vi "Configure Channel.vi"(0 "CS++Scope":refnum<class "CS++Scope.lvclass">, 1 "channel enabled (True)":bool=TRUE, 2 "channel name (\"CHANNEL1\")":string="CHANNEL1", 3 "probe attenuation (1:1.0)":dbl=1.0 format="%.3f", 4 "vertical offset (0.0 V)":dbl[unit] format="%.3f", 5 "error in (no error)":errorcluster, 6 "vertical coupling (DC)":i32(ring)=1 items=["AC", "DC", "GND"], 8 "vertical range (10.0 V)":dbl[unit]=10.0 format="%.3f") -> (14 "CS++Scope out":refnum<class "CS++Scope.lvclass">, 19 "error out":errorcluster)   [LabVIEW 2015, in "CS++Scope.lvlib" / "CS++Scope.lvclass"]
doc: "This VI configures the most commonly configured properties of the oscilloscope channel sub-system. These properties are the range, offset, coupling, probe attenuation, and whether the channel is enabled."
uses:
  CS++Scope.lvclass
  CSPP_Core/Classes/CS++ProcessVariables/ProcessVariable/PV.lvclass
  PV-Enum-n.ctl
  CSPP_Core/Classes/CS++ProcessVariables/ProcessVariable/PV.lvclass/PV.ctl
  CS++Scope.lvclass/CS++Scope.ctl
  CSPP_Core/Classes/CS++ProcessVariables/ProcessVariable/Write Data.vi
  CSPP_Core/Classes/CS++ProcessVariables/ProcessVariable/Write Timestamp.vi
  CSPP_Core/Classes/CS++ProcessVariables/ProcessVariable/Write Quality.vi
  CSPP_Core/Classes/CS++ProcessVariables/ProcessVariable/Write status.vi
  CSPP_Core/Classes/CS++ProcessVariables/PVConnection/PVConnection.lvclass
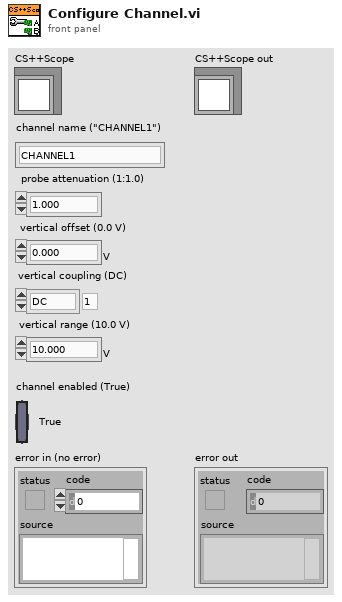
[diagram p1: front panel]
types:
  T1 = typedef "CS++Scope.lvlib/CS++Scope.lvclass/PV-Enum-n.ctl" = enum16{"InputImpedance", "MaxInputFrequency", "VerticalRange", "ProbeAttenuation", "VerticalOffset", "VerticalCoupling", "ChannelEnabled"}
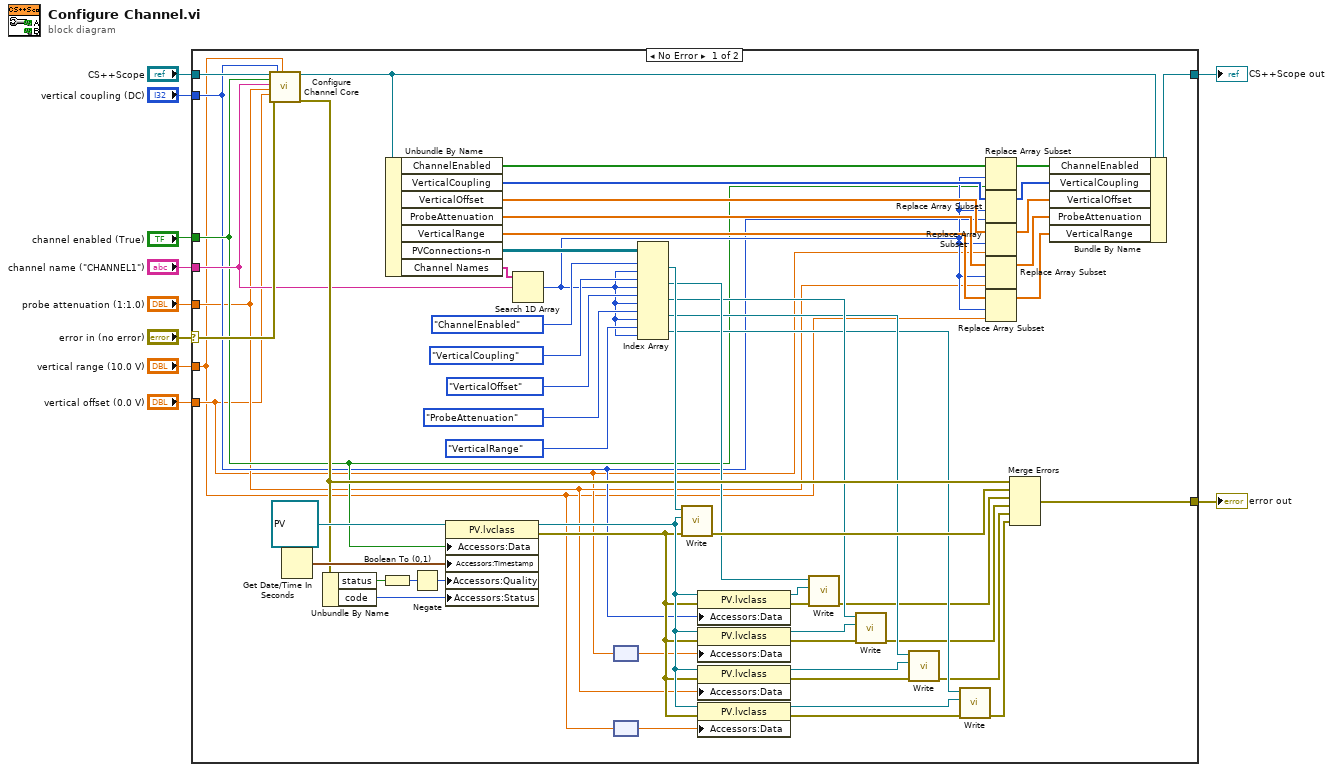
[diagram p0: block diagram]
diagram:
  n1 = case shown="No Error" "error in (no error)" {
    selector: "error in (no error)" -> [w55 w70]
    tunnel: [w29 w70] -> w9
    tunnel: [w56 w69] -> w2
    tunnel: "CS++Scope" -> [w57 w69]
    tunnel: "channel name (\"CHANNEL1\")" -> [w53 _]
    tunnel: "probe attenuation (1:1.0)" -> [w15 _]
    tunnel: "vertical range (10.0 V)" -> [w12 _]
    tunnel: "vertical offset (0.0 V)" -> [w14 _]
    tunnel: "channel enabled (True)" -> [w17 _]
    tunnel: "vertical coupling (DC)" -> [w16 _]
    frame No Error {
      n2 = call-dynamic "Configure Channel Core.vi"("CS++Scope"=w57, "channel enabled (True)"=w17, "channel name (\"CHANNEL1\")"=w53, "probe attenuation (1:1.0)"=w15, "vertical offset (0.0 V)"=w14, "error in (no error)"=w55, "vertical coupling (DC)"=w16, "vertical range (10.0 V)"=w12) -> ("CS++Scope out"=w68:refnum<class "CS++Scope.lvclass">, "error out"=w59:errorcluster)  [unwired: 10 in]
      n3 = Get Date/Time In Seconds() -> (seconds since 1Jan1904=w62:timestamp)
      n4 = Unbundle By Name(w59) -> ("status"=w65:bool, "code"=w66:i32)
      n5 = Boolean To (0,1)(Boolean=w65) -> (0, 1=w64:i16)
      n6 = Unbundle By Name(w68) -> ("ChannelEnabled"=w28:bool[], "VerticalCoupling"=w26:i32[], "VerticalOffset"=w24:dbl[unit][], "ProbeAttenuation"=w22:dbl[], "VerticalRange"=w19:dbl[unit][], "PVConnections-n"=w61:refnum<class "PVConnection.lvclass">[][], "Channel Names"=w54:string[])
      n7 = Negate(x=w64) -> (-x=w63:i16)
      n8 = property class="PV.lvclass"(reference=refnum<class "PV.lvclass"> refnum ("CS++ProcessVariables.lvlib:PV.lvclass"), "Accessors:Data"=w17, "Accessors:Timestamp"=w62, "Accessors:Quality"=w63, "Accessors:Status"=w66) -> (reference out=w36:refnum<class "PV.lvclass">, error out=w35:errorcluster)  [unwired: 1 in]
      n9 = Search 1D Array(1D array=w54, element=w53) -> (index of element=w18:i32)  [unwired: 1 in]
      n10 = node(w14) -> (w13:dbl)
      n11 = node(w12) -> (w11:dbl)
      n12 = Index Array(array=w61, index (row) #1=PV-Enum-n."ChannelEnabled" ("PV-Enum-n"), index (col) #1=w18, index (row) #2=PV-Enum-n."VerticalCoupling" ("PV-Enum-n"), index (col) #2=w18, index (row) #3=PV-Enum-n."VerticalOffset" ("PV-Enum-n"), index (col) #3=w18, index (row) #4=PV-Enum-n."ProbeAttenuation" ("PV-Enum-n"), index (col) #4=w18, index (row) #5=PV-Enum-n."VerticalRange" ("PV-Enum-n"), index (col) #5=w18) -> (element #1=w60:refnum<class "PVConnection.lvclass">, element #2=w45:refnum<class "PVConnection.lvclass">, element #3=w40:refnum<class "PVConnection.lvclass">, element #4=w39:refnum<class "PVConnection.lvclass">, element #5=w34:refnum<class "PVConnection.lvclass">)
      n13 = call "Write.vi"("error in (no error)"=w35, "PV"=w36, "PVConnection in"=w60) -> ("error out"=w58:errorcluster)  [unwired: 7 in, 1 out]
      n14 = property class="PV.lvclass"(reference=w36, error in=w35, "Accessors:Data"=w16) -> (reference out=w46:refnum<class "PV.lvclass">, error out=w47:errorcluster)
      n15 = property class="PV.lvclass"(reference=w36, error in=w35, "Accessors:Data"=w13) -> (reference out=w43:refnum<class "PV.lvclass">, error out=w44:errorcluster)
      n16 = property class="PV.lvclass"(reference=w36, error in=w35, "Accessors:Data"=w15) -> (reference out=w41:refnum<class "PV.lvclass">, error out=w42:errorcluster)
      n17 = property class="PV.lvclass"(reference=w36, error in=w35, "Accessors:Data"=w11) -> (reference out=w37:refnum<class "PV.lvclass">, error out=w38:errorcluster)
      n18 = call "Write.vi"("error in (no error)"=w47, "PV"=w46, "PVConnection in"=w45) -> ("error out"=w33:errorcluster)  [unwired: 7 in, 1 out]
      n19 = call "Write.vi"("error in (no error)"=w44, "PV"=w43, "PVConnection in"=w40) -> ("error out"=w32:errorcluster)  [unwired: 7 in, 1 out]
      n20 = call "Write.vi"("error in (no error)"=w42, "PV"=w41, "PVConnection in"=w39) -> ("error out"=w31:errorcluster)  [unwired: 7 in, 1 out]
      n21 = call "Write.vi"("error in (no error)"=w38, "PV"=w37, "PVConnection in"=w34) -> ("error out"=w30:errorcluster)  [unwired: 7 in, 1 out]
      n22 = Replace Array Subset(array=w28, new element=w17, index=w18) -> (w27:bool[])
      n23 = Replace Array Subset(array=w26, new element=w16, index=w18) -> (w25:i32[])
      n24 = Replace Array Subset(array=w24, new element=w14, index=w18) -> (w23:dbl[unit][])
      n25 = Replace Array Subset(array=w22, new element=w15, index=w18) -> (w21:dbl[])
      n26 = Replace Array Subset(array=w19, new element=w12, index=w18) -> (w20:dbl[unit][])
      n27 = Merge Errors(w59, w58, w33, w32, w31, w30) -> (w29:errorcluster)
      n28 = Bundle By Name(cluster=w68, "ChannelEnabled"=w27, "VerticalCoupling"=w25, "VerticalOffset"=w23, "ProbeAttenuation"=w21, "VerticalRange"=w20) -> (w56:refnum<class "CS++Scope.lvclass">)
    }
    frame Error {
    }
  }
  "error out" <- w9
  "CS++Scope out" <- w2
